vi "Enqueue Analysis.vi"(8 "error in (no error)":errorcluster, 10 "data":waveform(cdb), 11 "analysis queue":refnum<queue>) -> (0 "error out":errorcluster)   [LabVIEW 2021]
uses:
  Analysis Message.ctl
  Analysis Message with Waveform.ctl
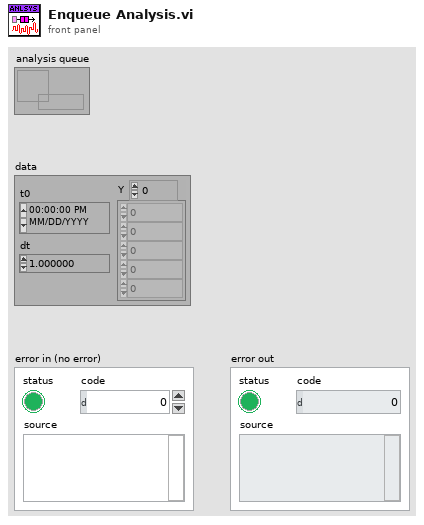
[diagram p1: front panel]
types:
  T1 = typedef "Analysis Message.ctl" = enum16{"Analyze", "Exit"}
  T2 = typedef "Analysis Message with Waveform.ctl" = cluster{"wfm dat":waveform(cdb), "msg":T1}
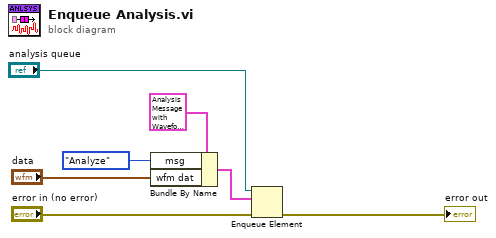
[diagram p0: block diagram]
diagram:
  n1 = Bundle By Name(cluster=T2 {"wfm dat"={"t0"=timestamp(0 s since 1904-01-01), "dt"=0.0, "Y"=[]}, "msg"=enum."Analyze"} ("element"), "msg"=Analysis_Message."Analyze", "wfm dat"="data") -> (w3:T2)
  n2 = Enqueue Element(queue="analysis queue", element=w3, error in (no error)="error in (no error)") -> (error out=→"error out":errorcluster)  [unwired: 1 in, 2 out]
